vi "Autonomous Independent.vi"() -> ()   [LabVIEW 2016]
doc: "This VI is called when autonomous begins, and will automatically be terminated when autonomous ends. You can carry out timed or sensor driven robot movement independently without needing to return to the caller."
panel:
  in  "Turn":dbl
  in  "DriveSpeed":dbl
  in  "TimeDrive":u32=2000
  # "Be sure to right-click and choose Data Operations>>Make Current Value default if you want to save the array values with the VI"
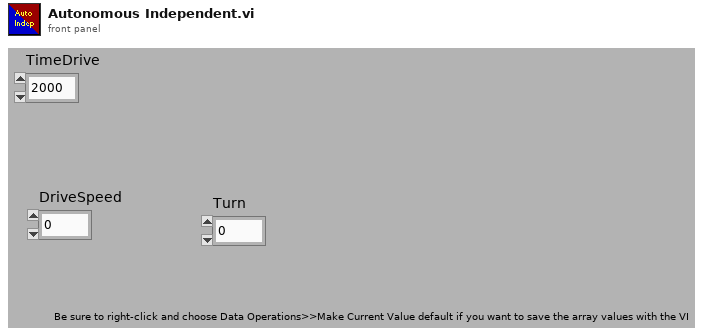
[diagram p1: front panel]
types:
  T1 = typedef "WPI_MotorControlDeviceRef.ctl" = cluster{"DeviceStatus":errorcluster, "Type":T2, "PWM":cluster{"PWM Channel":T3, "DeadBand":T4}, "CAN":cluster{"Device Number":u8, "SetOutput VI Ref":variant, "GetOutput VI Ref":variant, "Enable VI Ref":variant, "Disable VI Ref":variant, "Data":variant}, "Invert":bool}
  T2 = typedef "WPI_MotorControlType.ctl" = enum16{"PWM", "CAN"}
  T3 = typedef "FPGA_DIOPWMChannel.ctl" = enum8{"PWM 0", "PWM 1", "PWM 2", "PWM 3", "PWM 4", "PWM 5", "PWM 6", "PWM 7", "PWM 8", "PWM 9", "PWM MXP 0", "PWM MXP 1", "PWM MXP 2", "PWM MXP 3", "PWM MXP 4", "PWM MXP 5", "PWM MXP 6", "PWM MXP 7", "PWM MXP 8", "PWM MXP 9", "Invalid"}
  T4 = typedef "WPI_PWMDeadband.ctl" = cluster{"Name":string, "maxPositivePwm":i32, "minPositivePwm":i32, "centerPwm":i32, "maxNegativePwm":i32, "minNegativePwm":i32, "angularRange":u16}
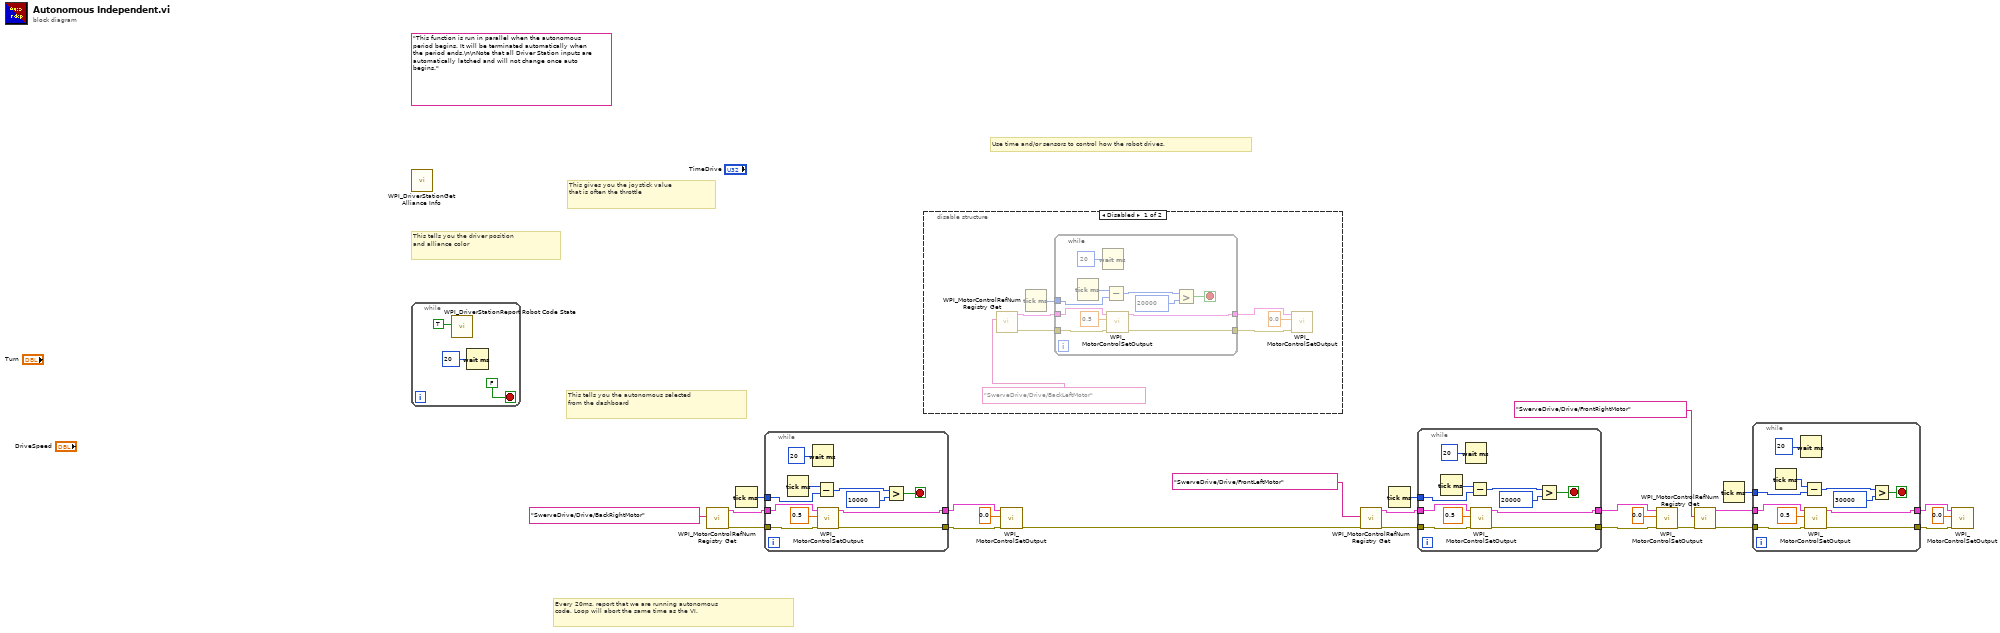
[diagram p0: block diagram]
diagram:
  (unwired) "This function is run in parallel when the autonomous period begins. It will be terminated automatically when the period ends.\n\nNote that all Driver Station inputs are automatically latched and will not change once auto begins."
  # "Every 20ms, report that we are running autonomous\ncode. Loop will abort the same time as the VI."
  # "This tells you the autonomous selected\nfrom the dashboard"
  # "This gives you the joystick value\nthat is often the throttle"
  # "Use time and/or sensors to control how the robot drives."
  # "This tells you the driver position\nand alliance color"
  n1 = call <vilib>:"WPI_DriverStationGet Alliance Info.vi"() -> ()  [unwired: 12 out]
  n2 = while {
    stop <- FALSE stop-if-true
    n3 = call <vilib>:"WPI_DriverStationReport Robot Code State.vi"("Autonomous"=TRUE) -> ()  [unwired: 10 in, 1 out]
    n4 = Wait (ms)(milliseconds to wait=u32 20) -> ()  [unwired: 1 out]
  }
  n5 = call <vilib>:"WPI_MotorControlRefNum Registry Get.vi"("refnum name"="SwerveDrive/Drive/BackRightMotor") -> ("error out"=w15:errorcluster, "MotorControlDevRef"=w14:T1)  [unwired: 9 in]
  n6 = Tick Count (ms)() -> (millisecond timer value=w12:u32)
  n7 = while {
    tunnel: w14 -> [w35]
    tunnel: w12 -> [w33]
    tunnel: [w36] -> w16
    tunnel: w15 -> [w34]
    tunnel: [w37] -> w11
    stop <- w30 stop-if-true
    n8 = Tick Count (ms)() -> (millisecond timer value=w31:u32)
    n9 = Wait (ms)(milliseconds to wait=u32 20) -> ()  [unwired: 1 out]
    n10 = Subtract(x=w31, y=w33) -> (x-y=w32:u32)
    n11 = call <vilib>:"WPI_MotorControlSetOutput.vi"("error in (no error)"=w34, "Output"=0.5, "MotorControlDevRef"=w35) -> ("error out"=w37:errorcluster, "MotorControlDevRef"=w36:T1)  [unwired: 6 in, 1 out]
    n12 = Greater?(x=w32, y=u32 10000) -> (0:w30:bool)
  }
  n13 = disable-structure shown="Disabled" {
    frame Disabled {
      n14 = call <vilib>:"WPI_MotorControlRefNum Registry Get.vi"("refnum name"="SwerveDrive/Drive/BackLeftMotor") -> ("error out"=w43:errorcluster, "MotorControlDevRef"=w42:T1)  [unwired: 9 in]
      n15 = Tick Count (ms)() -> (millisecond timer value=w44:u32)
      n16 = while {
        tunnel: w42 -> [w49]
        tunnel: w44 -> [w55]
        tunnel: [w46] -> w39
        tunnel: w43 -> [w48]
        tunnel: [w47] -> w40
        stop <- w52 stop-if-true
        n17 = Tick Count (ms)() -> (millisecond timer value=w53:u32)
        n18 = Wait (ms)(milliseconds to wait=u32 20) -> ()  [unwired: 1 out]
        n19 = Subtract(x=w53, y=w55) -> (x-y=w54:u32)
        n20 = call <vilib>:"WPI_MotorControlSetOutput.vi"("error in (no error)"=w48, "Output"=0.5, "MotorControlDevRef"=w49) -> ("error out"=w47:errorcluster, "MotorControlDevRef"=w46:T1)  [unwired: 6 in, 1 out]
        n21 = Greater?(x=w54, y=u32 20000) -> (0:w52:bool)
      }
      n22 = call <vilib>:"WPI_MotorControlSetOutput.vi"("error in (no error)"=w40, "Output"=0.0, "MotorControlDevRef"=w39) -> ()  [unwired: 6 in, 3 out]
    }
    frame Enabled {
    }
  }
  n23 = call <vilib>:"WPI_MotorControlSetOutput.vi"("error in (no error)"=w11, "Output"=0.0, "MotorControlDevRef"=w16) -> ("error out"=w17:errorcluster)  [unwired: 6 in, 2 out]
  n24 = call <vilib>:"WPI_MotorControlRefNum Registry Get.vi"("error in (no error)"=w17, "refnum name"="SwerveDrive/Drive/FrontLeftMotor") -> ("error out"=w19:errorcluster, "MotorControlDevRef"=w18:T1)  [unwired: 8 in]
  n25 = Tick Count (ms)() -> (millisecond timer value=w8:u32)
  n26 = while {
    tunnel: w18 -> [w63]
    tunnel: w8 -> [w62]
    tunnel: [w65] -> w7
    tunnel: w19 -> [w64]
    tunnel: [w66] -> w20
    stop <- w59 stop-if-true
    n27 = Tick Count (ms)() -> (millisecond timer value=w60:u32)
    n28 = Wait (ms)(milliseconds to wait=u32 20) -> ()  [unwired: 1 out]
    n29 = Subtract(x=w60, y=w62) -> (x-y=w61:u32)
    n30 = call <vilib>:"WPI_MotorControlSetOutput.vi"("error in (no error)"=w64, "Output"=0.5, "MotorControlDevRef"=w63) -> ("error out"=w66:errorcluster, "MotorControlDevRef"=w65:T1)  [unwired: 6 in, 1 out]
    n31 = Greater?(x=w61, y=u32 20000) -> (0:w59:bool)
  }
  n32 = call <vilib>:"WPI_MotorControlSetOutput.vi"("error in (no error)"=w20, "Output"=0.0, "MotorControlDevRef"=w7) -> ("error out"=w21:errorcluster)  [unwired: 6 in, 2 out]
  n33 = call <vilib>:"WPI_MotorControlRefNum Registry Get.vi"("error in (no error)"=w21, "refnum name"="SwerveDrive/Drive/FrontRightMotor") -> ("error out"=w23:errorcluster, "MotorControlDevRef"=w22:T1)  [unwired: 8 in]
  n34 = Tick Count (ms)() -> (millisecond timer value=w1:u32)
  n35 = while {
    tunnel: w22 -> [w77]
    tunnel: w1 -> [w72]
    tunnel: [w74] -> w3
    tunnel: w23 -> [w76]
    tunnel: [w75] -> w4
    stop <- w69 stop-if-true
    n36 = Tick Count (ms)() -> (millisecond timer value=w70:u32)
    n37 = Wait (ms)(milliseconds to wait=u32 20) -> ()  [unwired: 1 out]
    n38 = Subtract(x=w70, y=w72) -> (x-y=w71:u32)
    n39 = call <vilib>:"WPI_MotorControlSetOutput.vi"("error in (no error)"=w76, "Output"=0.5, "MotorControlDevRef"=w77) -> ("error out"=w75:errorcluster, "MotorControlDevRef"=w74:T1)  [unwired: 6 in, 1 out]
    n40 = Greater?(x=w71, y=u32 30000) -> (0:w69:bool)
  }
  n41 = call <vilib>:"WPI_MotorControlSetOutput.vi"("error in (no error)"=w4, "Output"=0.0, "MotorControlDevRef"=w3) -> ()  [unwired: 6 in, 3 out]
